vi "SystemLink_Write.vi"(8 "String":string, 9 "Numeric":dbl, 11 "Thingworx":T1(xcontrol)) -> ()   [LabVIEW 2019]
uses:
  _Subs/SL_XControl.xctl
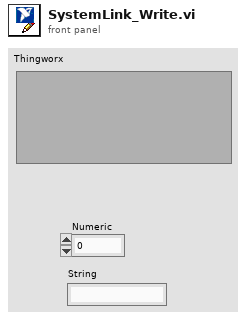
[diagram p1: front panel]
types:
  T1 = cluster{"Tag":string, "Type":string, "Data":string}
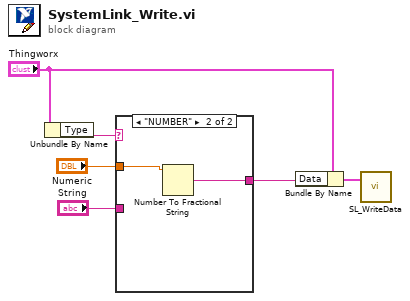
[diagram p0: block diagram]
diagram:
  n1 = Unbundle By Name("Thingworx") -> ("Type"=w5:string)
  n2 = case shown="\"NUMBER\"" w5 {
    tunnel: "Numeric" -> [_ w9]
    tunnel: [w7 w8] -> w4
    tunnel: "String" -> [w7 _]
    frame Default {
    }
    frame "NUMBER" {
      n3 = Number To Fractional String(number=w9) -> (F-format string=w8:string)  [unwired: 3 in]
    }
  }
  n4 = Bundle By Name(cluster="Thingworx", "Data"=w4) -> (w1:T1)
  n5 = call "SL_WriteData.vi"("Tag"=w1) -> ()  [unwired: 11 in]
